vi "parse core.vi"(11 "URL":string) -> (0 "query":string, 1 "path":string, 2 "port":string, 3 "host":string, 4 "password":string, 5 "username":string, 6 "fragment":string, 7 "scheme":string)   [LabVIEW 2013, in "uniform resource locator.lvlib"]
uses:
  uniform resource locator.lvlib
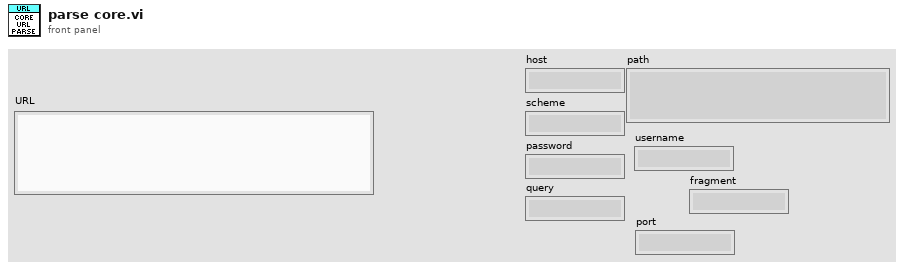
[diagram p1: front panel]
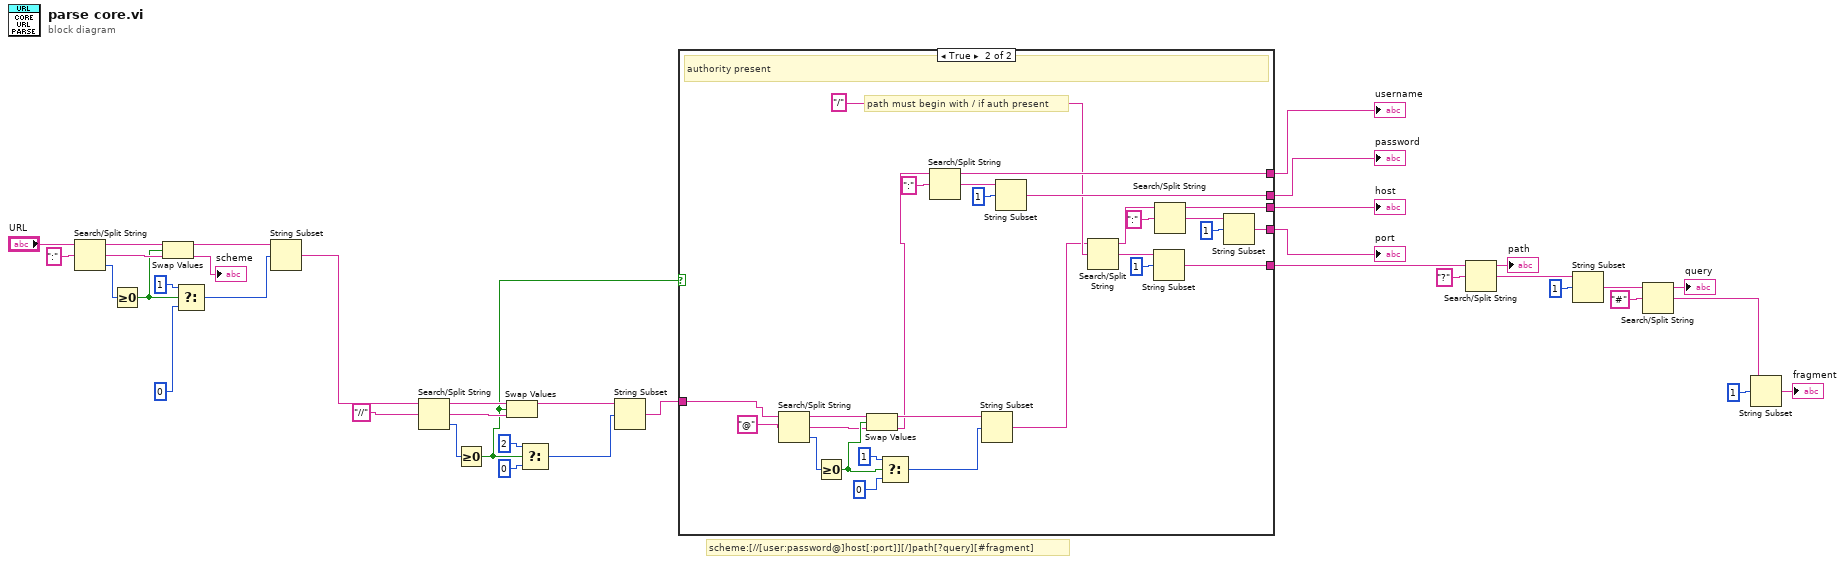
[diagram p0: block diagram]
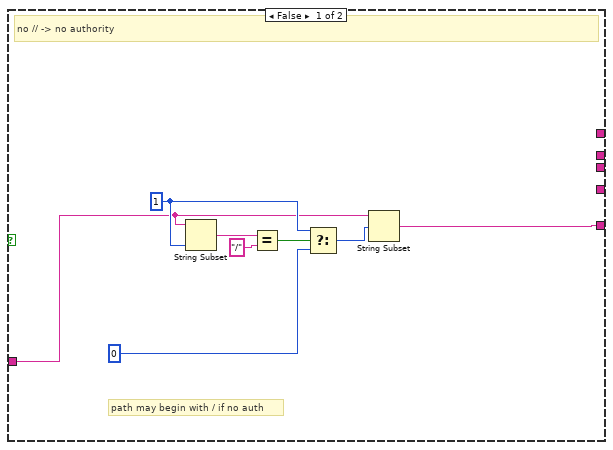
[diagram p2: hidden frame]
diagram:
  # "scheme:[//[user:password@]host[:port]][/]path[?query][#fragment]"
  n1 = Search/Split String(string="URL", search string/char (-)=":" ("regular expression")) -> (substring before match=w19:string, match + rest of string=w18:string, offset of match=w20:i32)  [unwired: 1 in]
  n2 = Greater Or Equal To 0?(x=w20) -> (x >= 0?=w15:bool)
  n3 = Swap Values(12:w19, 13:w15, 14:w18) -> (1:w16:string, 3:→"scheme":string)
  n4 = Select(t=1 ("offset (0)"), s=w15, f=0 ("offset (0)")) -> (s? t:f=w12:i32)
  n5 = String Subset(string=w16, offset (0)=w12) -> (substring=w5:string)  [unwired: 1 in]
  n6 = Search/Split String(string=w5, search string/char (-)="//" ("regular expression")) -> (substring before match=w6:string, match + rest of string=w7:string, offset of match=w3:i32)  [unwired: 1 in]
  n7 = Greater Or Equal To 0?(x=w3) -> (x >= 0?=w1:bool)
  n8 = Swap Values(12:w6, 13:w1, 14:w7) -> (1:w8:string)  [unwired: 1 out]
  n9 = Select(t=2 ("offset (0)"), s=w1, f=0 ("offset (0)")) -> (s? t:f=w11:i32)
  n10 = String Subset(string=w8, offset (0)=w11) -> (substring=w2:string)  [unwired: 1 in]
  n11 = case shown="True" w1 {
    tunnel: [_ w65] -> w35
    tunnel: [w43 w68] -> w29
    tunnel: [_ w72] -> w34
    tunnel: [_ w71] -> w33
    tunnel: [_ w61] -> w21
    tunnel: w2 -> [w38 w52]
    frame False {
      w41 = 1 ("length (rest)")
      # "path may begin with / if no auth"
      # "no // -> no authority"
      n12 = String Subset(string=w38, length (rest)=w41) -> (substring=w45:string)  [unwired: 1 in]
      n13 = Equal?(x=w45, y="/" ("regular expression")) -> (x = y?=w42:bool)
      n14 = Select(t=w41, s=w42, f=0) -> (s? t:f=w39:i32)
      n15 = String Subset(string=w38, offset (0)=w39) -> (substring=w43:string)  [unwired: 1 in]
    }
    frame True {
      # "path must begin with / if auth present"
      # "authority present"
      n16 = Search/Split String(string=w52, search string/char (-)="@" ("regular expression")) -> (substring before match=w58:string, match + rest of string=w57:string, offset of match=w59:i32)  [unwired: 1 in]
      n17 = Greater Or Equal To 0?(x=w59) -> (x >= 0?=w60:bool)
      n18 = Swap Values(12:w58, 13:w60, 14:w57) -> (1:w56:string, 3:w46:string)
      n19 = Select(t=1 ("offset (0)"), s=w60, f=0 ("offset (0)")) -> (s? t:f=w53:i32)
      n20 = Search/Split String(string=w46, search string/char (-)=":" ("regular expression")) -> (substring before match=w72:string, match + rest of string=w49:string)  [unwired: 1 in, 1 out]
      n21 = String Subset(string=w56, offset (0)=w53) -> (substring=w50:string)  [unwired: 1 in]
      n22 = String Subset(string=w49, offset (0)=1) -> (substring=w71:string)  [unwired: 1 in]
      n23 = Search/Split String(string=w50, search string/char (-)="/" ("regular expression")) -> (substring before match=w63:string, match + rest of string=w70:string)  [unwired: 1 in, 1 out]
      n24 = String Subset(string=w70, offset (0)=1) -> (substring=w68:string)  [unwired: 1 in]
      n25 = Search/Split String(string=w63, search string/char (-)=":" ("regular expression")) -> (substring before match=w65:string, match + rest of string=w66:string)  [unwired: 1 in, 1 out]
      n26 = String Subset(string=w66, offset (0)=1) -> (substring=w61:string)  [unwired: 1 in]
    }
  }
  "host" <- w35
  "username" <- w34
  "password" <- w33
  "port" <- w21
  n27 = Search/Split String(string=w29, search string/char (-)="?" ("regular expression")) -> (substring before match=→"path":string, match + rest of string=w30:string)  [unwired: 1 in, 1 out]
  n28 = String Subset(string=w30, offset (0)=1) -> (substring=w24:string)  [unwired: 1 in]
  n29 = Search/Split String(string=w24, search string/char (-)="#" ("regular expression")) -> (substring before match=→"query":string, match + rest of string=w26:string)  [unwired: 1 in, 1 out]
  n30 = String Subset(string=w26, offset (0)=1) -> (substring=→"fragment":string)  [unwired: 1 in]
